vi "Write to excel.vi"(0 "Mapp":path, 1 "Filnamn":string, 2 "Boolean":bool, 3 "Spänning":dbl, 4 "Ström":dbl, 8 "Ytresistivitet":dbl, 9 "Ytresistans":dbl) -> (6 "error out":errorcluster)   [LabVIEW 2024]
uses:
  <vilib>/express/express shared/transition.llb/Dynamic To Waveform Array.vi
  <vilib>/express/express signal manip/GetorSetDDTAttributes/Set DDT Attributes/SetT0.vi
  <vilib>/express/express shared/transition.llb/Waveform Array To Dynamic.vi
  <vilib>/express/express signal manip/GetorSetDDTAttributes/Set DDT Attributes/Set DDT Properties.xnode
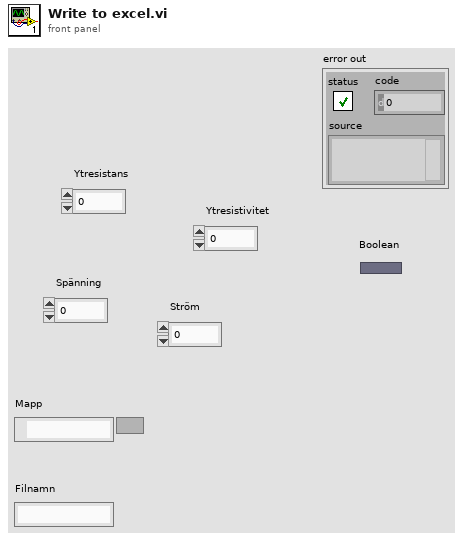
[diagram p1: front panel]
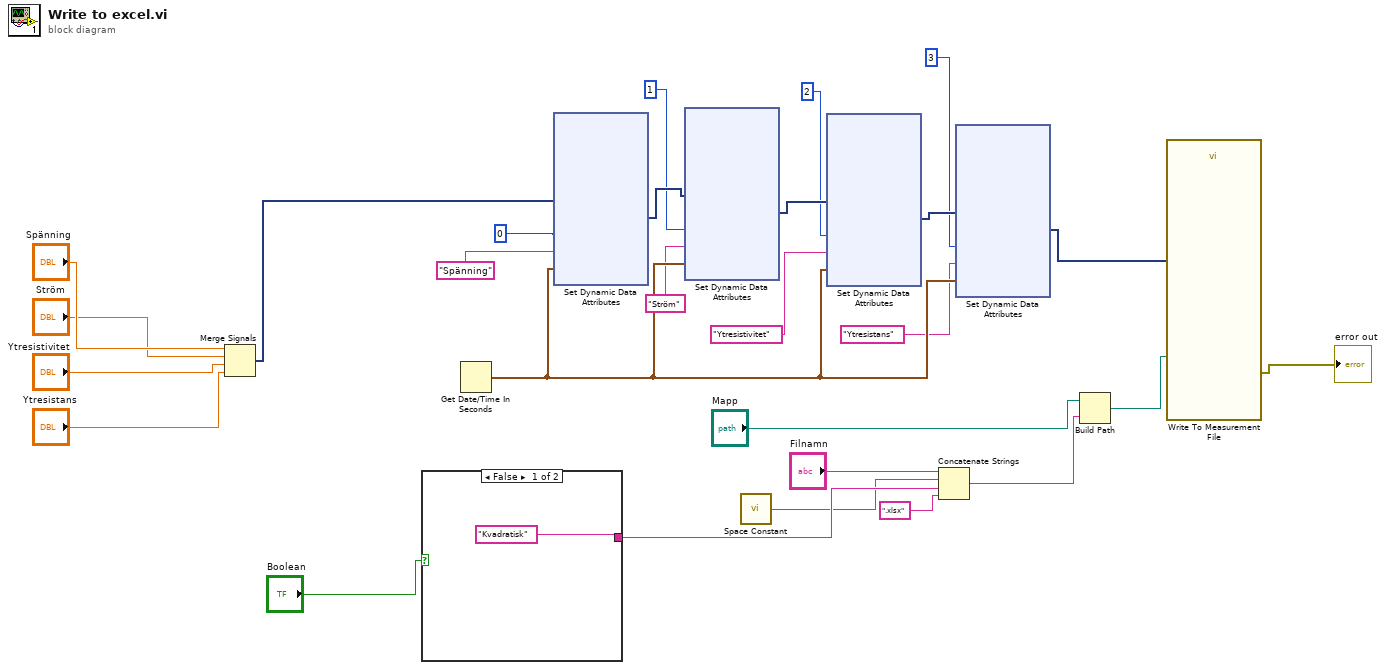
[diagram p0: block diagram]
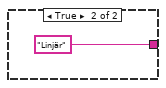
[diagram p2: hidden frame]
diagram:
  n1 = Merge Signals("Spänning", "Ström", "Ytresistivitet", "Ytresistans") -> (w23:dynamicdata)
  n2 = case shown="False" "Boolean" {
    tunnel: ["Kvadratisk" "Linjär"] -> w3
    frame False {
    }
    frame True {
    }
  }
  n3 = Get Date/Time In Seconds() -> (seconds since 1Jan1904=w21:timestamp)
  n4 = xnode "Set Dynamic Data Attributes"("Signals In"=w23, "Signal Index"=0, "Signal Name"="Spänning", "Timestamp"=w21) -> ("Signals Out"=w16:dynamicdata)  [unwired: 1 in, 1 out]
  n5 = xnode "Set Dynamic Data Attributes"("Signals In"=w16, "Signal Index"=1, "Signal Name"="Ström", "Timestamp"=w21) -> ("Signals Out"=w15:dynamicdata)  [unwired: 1 in, 1 out]
  n6 = call <vilib>:"Space Constant.vi"() -> ("String"=w2:string)
  n7 = xnode "Set Dynamic Data Attributes"("Signals In"=w15, "Signal Index"=2, "Signal Name"="Ytresistivitet", "Timestamp"=w21) -> ("Signals Out"=w14:dynamicdata)  [unwired: 1 in, 1 out]
  n8 = Concatenate Strings("Filnamn", w2, w3, ".xlsx" ("string")) -> (w11:string)
  n9 = xnode "Set Dynamic Data Attributes"("Signals In"=w14, "Signal Index"=3, "Signal Name"="Ytresistans", "Timestamp"=w21) -> ("Signals Out"=w13:dynamicdata)  [unwired: 1 in, 1 out]
  n10 = Build Path(base path="Mapp", name or relative path=w11) -> (appended path=w7:path)
  n11 = call "Write To Measurement File"("Signals"=w13, "Filename"=w7) -> ("error out"=→"error out":errorcluster)  [unwired: 15 in, 2 out]
